vi "overlay_rectangle_thc.vi"(0 "Image In":T2, 1 "Thickness":i32, 2 "Rectangle":T1, 3 "Error In":errorcluster, 4 "Color":u32(colorbox)) -> (5 "Image Out":T2, 6 "Error Out":errorcluster)   [LabVIEW 2019]
uses:
  <vilib>/vision/Image Controls.llb/IMAQ Image.ctl
panel:
  # "Thanks to Paul M. for providing this VI, which has been modified to better suit the needs of this project. \nMore info here: https://forums.ni.com/t5/Example-Code/Adjustable-Rectangular-Overlay-Line-Thickness/ta-p/3509087?profile.language=en"
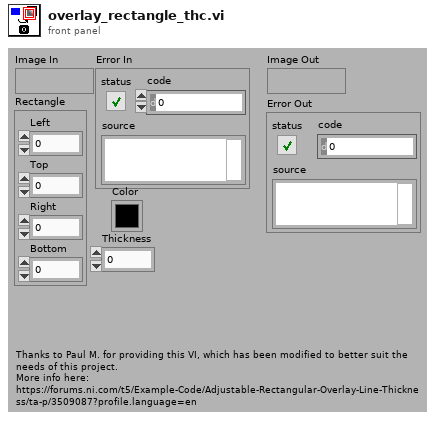
[diagram p1: front panel]
types:
  T1 = cluster{"Left":i32, "Top":i32, "Right":i32, "Bottom":i32}
  T2 = typedef "IMAQ Image.ctl" = refnum<image>
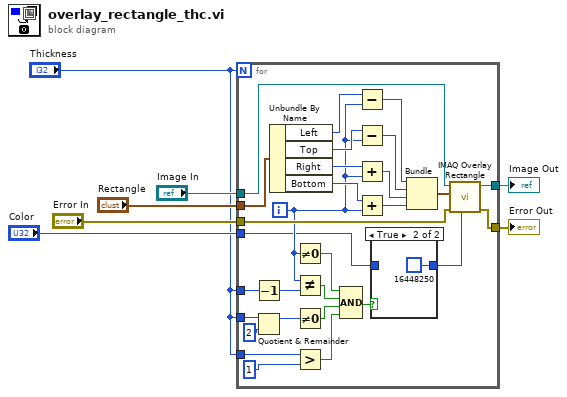
[diagram p0: block diagram]
diagram:
  n1 = for {
    N: "Thickness" -> [_]
    tunnel: "Image In" -> [w36]
    tunnel: "Error In" -> [w35]
    tunnel: [w34] -> w4
    tunnel: "Rectangle" -> [w33]
    tunnel: "Color" -> [w9]
    tunnel: [w23] -> w3
    tunnel: "Thickness" -> [w22]
    tunnel: "Thickness" -> [w19]
    tunnel: "Thickness" -> [w16]
    i -> [w17]
    n2 = Decrement(x=w16) -> (x-1=w15:i32)
    n3 = Quotient & Remainder(x=w22, y=2) -> (x-y*floor(x/y)=w20:i32)  [unwired: 1 out]
    n4 = Unbundle By Name(w33) -> ("Left"=w32:i32, "Top"=w31:i32, "Right"=w29:i32, "Bottom"=w30:i32)
    n5 = Not Equal To 0?(x=w17) -> (x != 0?=w14:bool)
    n6 = Not Equal?(x=w17, y=w15) -> (x != y?=w13:bool)
    n7 = Not Equal To 0?(x=w20) -> (x != 0?=w12:bool)
    n8 = Greater?(x=w19, y=1) -> (0:w11:bool)
    n9 = Compound Arithmetic op=AND(w14, w13, w12, w11) -> (w10:bool)
    n10 = Subtract(x=w32, y=w17) -> (x-y=w28:i32)
    n11 = Subtract(x=w31, y=w17) -> (x-y=w27:i32)
    n12 = Add(x=w29, y=w17) -> (x+y=w26:i32)
    n13 = Add(x=w30, y=w17) -> (x+y=w25:i32)
    n14 = case shown="True" w10 {
      tunnel: w9 -> [w37 _]
      tunnel: [w37 u32 16448250 ("Color")] -> w8
      frame False {
      }
      frame True {
      }
    }
    n15 = Bundle(w28, w27, w26, w25) -> (w24:cluster{i32, i32, i32, i32})  [unwired: 1 in]
    n16 = call "IMAQ Overlay Rectangle"("Color"=w8, "error in (no error)"=w35, "Rectangle"=w24, "Image"=w36) -> ("error out"=w23:errorcluster, "Image Out"=w34:T2)  [unwired: 6 in]
  }
  "Image Out" <- w4
  "Error Out" <- w3
